vi "ini_build_objects_list.vi"(8 "error in":errorcluster, 9 "VI rel path (empty)":string, 10 "VI name (empty)":string, 11 "objects":refnum<vi>[](array[refnum])) -> (0 "error out":errorcluster, 3 "objects list":string)   [LabVIEW 2020]
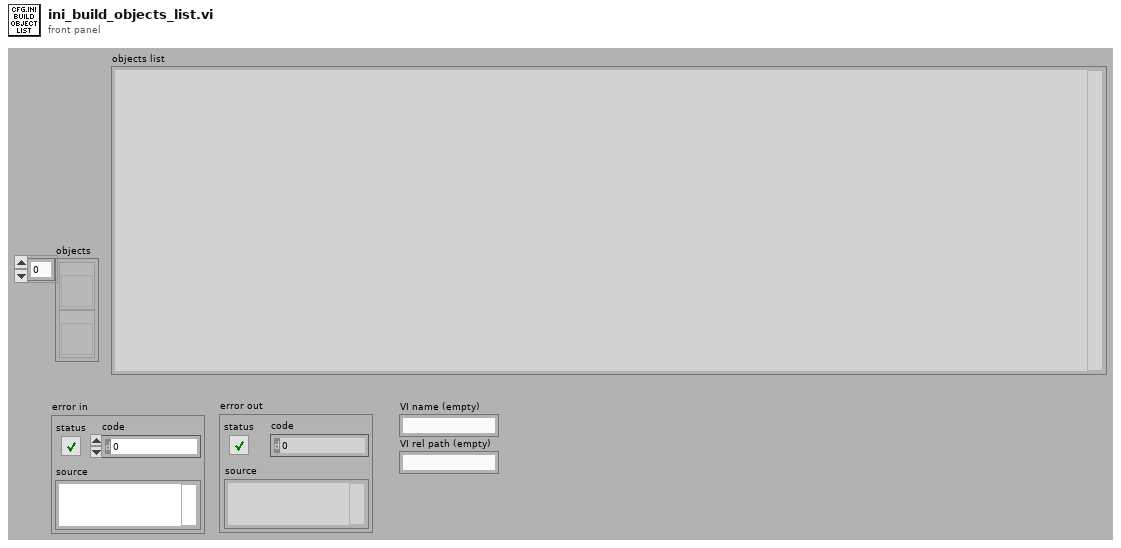
[diagram p1: front panel]
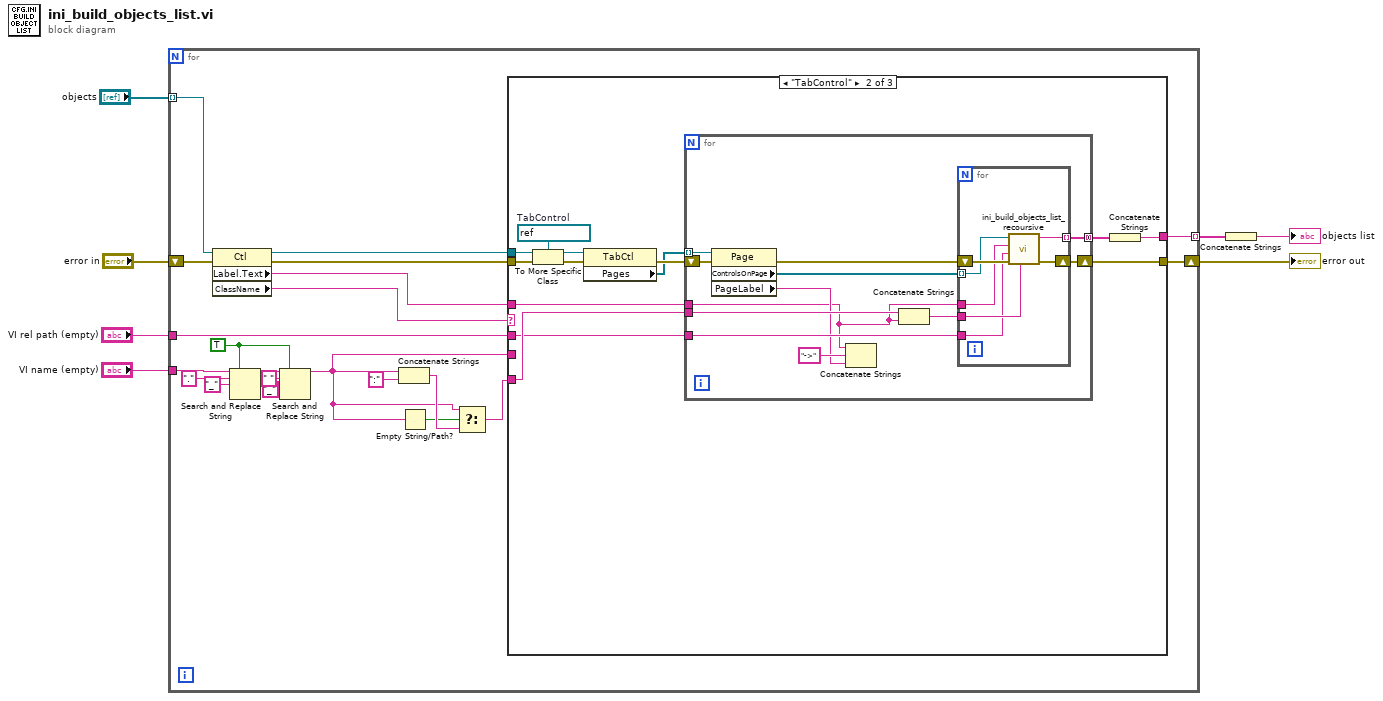
[diagram p0: block diagram]
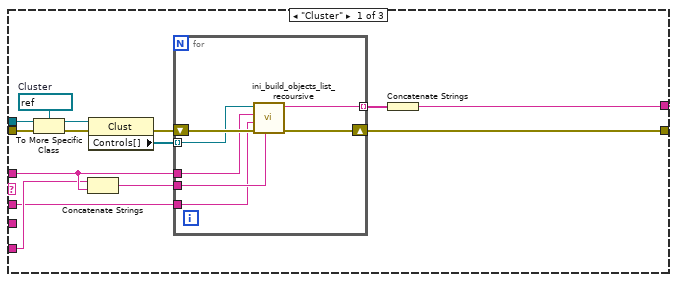
[diagram p2: hidden frame]
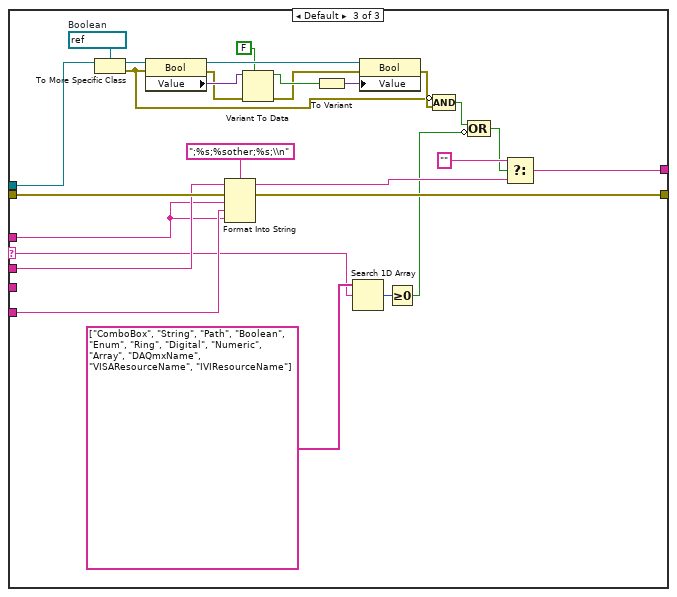
[diagram p3: hidden frame]
diagram:
  n1 = for {
    tunnel: "objects" -> [w27] mode=indexing
    shift-right: [w23] -> w5
    shift-left: "error in" -> [w28]
    tunnel: [w22] -> w4 mode=indexing
    tunnel: "VI name (empty)" -> [w16]
    tunnel: "VI rel path (empty)" -> [w13]
    w8 = TRUE ("ignore case? (F)")
    n2 = property class="Ctl"(reference=w27, error in=w28) -> (reference out=w25:refnum<vi>, error out=w24:errorcluster, "Label.Text"=w15:string, "ClassName"=w26:string)
    n3 = Search and Replace String(replace all?=w8, input string=w16, search string="." ("substring (\"\")"), replace string="_" ("replace string (\"\")")) -> (result string=w12:string)  [unwired: 4 in, 3 out]
    n4 = Search and Replace String(replace all?=w8, input string=w12, search string=" ", replace string="_" ("replace string (\"\")")) -> (result string=w11:string)  [unwired: 4 in, 3 out]
    n5 = Concatenate Strings(w11, ":" ("string")) -> (w18:string)
    n6 = Empty String/Path?(string/path=w11) -> (empty?=w14:bool)
    n7 = Select(t=w11, s=w14, f=w18) -> (s? t:f=w17:string)
    n8 = case shown="\"TabControl\"" w26 {
      selector: w26 -> [_ _ w82]
      tunnel: w25 -> [w42 w62 w104]
      tunnel: w24 -> [w40 w60 w107]
      tunnel: w15 -> [w31 w51 w86]
      tunnel: [w34 w56 w103] -> w22
      tunnel: [w33 w55 w98] -> w23
      tunnel: w17 -> [w30 w54 w105]
      tunnel: w13 -> [w29 w53 w106]
      tunnel: w11 -> [_ _ _]
      frame "Cluster" {
        w41 = refnum<vi> refnum  # Cluster
        n9 = To More Specific Class(target class=w41, reference=w42, error in=w40) -> (specific class reference=w38:refnum<vi>, error out=w39:errorcluster)
        n10 = Concatenate Strings(w30, w31) -> (w32:string)
        n11 = property class="Clust"(reference=w38, error in=w39) -> (error out=w36:errorcluster, "Controls[]"=w37:refnum<vi>[])  [unwired: 1 out]
        n12 = for {
          tunnel: w37 -> [w48] mode=indexing
          shift-right: [w47] -> w33
          shift-left: w36 -> [w49]
          tunnel: [w46] -> w35 mode=indexing
          tunnel: w31 -> [w45]
          tunnel: w32 -> [w44]
          tunnel: w29 -> [w43]
          n13 = call "ini_build_objects_list_recoursive.vi"("base cluster"=w44, "error in"=w49, "owning vi rel path"=w43, "owner chain (empty)"=w45, "Ctl Refnum"=w48) -> ("error out"=w47:errorcluster, "item"=w46:string)  [unwired: 5 in]
        }
        n14 = Concatenate Strings(w35) -> (w34:string)
      }
      frame "TabControl" {
        w61 = refnum<vi> refnum  # TabControl
        n15 = To More Specific Class(target class=w61, reference=w62, error in=w60) -> (specific class reference=w58:refnum<vi>, error out=w59:errorcluster)
        n16 = property class="TabCtl"(reference=w58, error in=w59) -> (error out=w52:errorcluster, "Pages"=w50:refnum<vi>[])  [unwired: 1 out]
        n17 = for {
          tunnel: [w74] -> w57 mode=concatenating
          tunnel: w54 -> [w72]
          tunnel: w53 -> [w71]
          tunnel: w51 -> [w63]
          shift-right: [w73] -> w55
          shift-left: w52 -> [w70]
          tunnel: w50 -> [w64] mode=indexing
          n18 = property class="Page"(reference=w64, error in=w70) -> (error out=w68:errorcluster, "ControlsOnPage"=w69:refnum<vi>[], "PageLabel"=w65:string)  [unwired: 1 out]
          n19 = Concatenate Strings(w63, "->" ("string"), w65) -> ()  [unwired: 1 out]
          n20 = Concatenate Strings(w72, w63) -> (w67:string)
          n21 = for {
            tunnel: w69 -> [w80] mode=indexing
            shift-right: [w79] -> w73
            shift-left: w68 -> [w81]
            tunnel: [w78] -> w74 mode=indexing
            tunnel: w63 -> [w77]
            tunnel: w67 -> [w76]
            tunnel: w71 -> [w75]
            n22 = call "ini_build_objects_list_recoursive.vi"("base cluster"=w76, "error in"=w81, "owning vi rel path"=w75, "owner chain (empty)"=w77, "Ctl Refnum"=w80) -> ("error out"=w79:errorcluster, "item"=w78:string)  [unwired: 5 in]
          }
        }
        n23 = Concatenate Strings(w57) -> (w56:string)
      }
      frame Default {
        w99 = refnum<vi> refnum  # Boolean
        n24 = To More Specific Class(target class=w99, reference=w104) -> (specific class reference=w100:refnum<vi>, error out=w93:errorcluster)  [unwired: 1 in]
        n25 = property class="Bool"(reference=w100, error in=w93) -> (reference out=w97:refnum<vi>, error out=w89:errorcluster, "Value"=w95:variant)
        n26 = Format Into String(format string=";%s;%sother;%s;\\n", initial string=w106, error in=w107, w86, w105, w86) -> (resulting string=w102:string, error out=w98:errorcluster)
        n27 = Variant To Data(error in=w89, type=FALSE, Variant=w95) -> (data=w94:bool, error out=w92:errorcluster)
        n28 = To Variant(anything=w94) -> (Variant=w90:variant)
        n29 = Search 1D Array(1D array=string[] ["ComboBox", "String", "Path", "Boolean", "Enum", "Ring", "Digital", "Numeric", "Array", "DAQmxName", "VISAResourceName", "IVIResourceName"], element=w82) -> (index of element=w87:i32)  [unwired: 1 in]
        n30 = property class="Bool"(reference=w97, error in=w92, "Value"=w90) -> (error out=w96:errorcluster)  [unwired: 1 out]
        n31 = Greater Or Equal To 0?(x=w87) -> (x >= 0?=w83:bool)
        n32 = Compound Arithmetic op=AND(invert w93, w96) -> (w85:bool)
        n33 = Compound Arithmetic op=OR(w85, invert w83) -> (w84:bool)
        n34 = Select(t="", s=w84, f=w102) -> (s? t:f=w103:string)
      }
    }
  }
  "error out" <- w5
  n35 = Concatenate Strings(w4) -> (→"objects list":string)
